vi "HTTP.StringToArray.vi"(7 "Separator":string=",", 10 "string":string) -> (2 "Array":string[](array[string]))   [LabVIEW 2013, in "Connection.WS_GOSPL.lvlib" / "Connection.WS.lvclass"]
uses:
  Connection.WS.lvclass
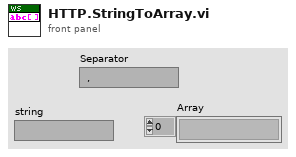
[diagram p1: front panel]
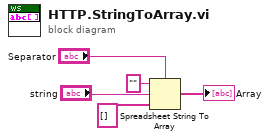
[diagram p0: block diagram]
diagram:
  n1 = Spreadsheet String To Array(delimiter (Tab)="Separator", format string="", spreadsheet string="string", array type (2D Dbl)=string[] []) -> (array=→"Array":string[])
